vi "Thread Loop.vi"(8 "error in (no error)":errorcluster, 11 "Vehicle Position Simulation in":refnum<class "Vehicle Position Simulation.lvclass">) -> (0 "error out":errorcluster, 3 "Vehicle Position Simulation out":refnum<class "Vehicle Position Simulation.lvclass">)   [LabVIEW 2012, in "Vehicle Position Simulation.lvlib" / "Vehicle Position Simulation.lvclass"]
uses:
  Vehicle Position Simulation.lvclass
  Thread/Thread.lvclass
panel:
  in  "Horizontal Pointer Slide":dbl(slide) scale=0.0..4.0
  # "[Covers: UI4]"
  # "[Covers: UI4A]"
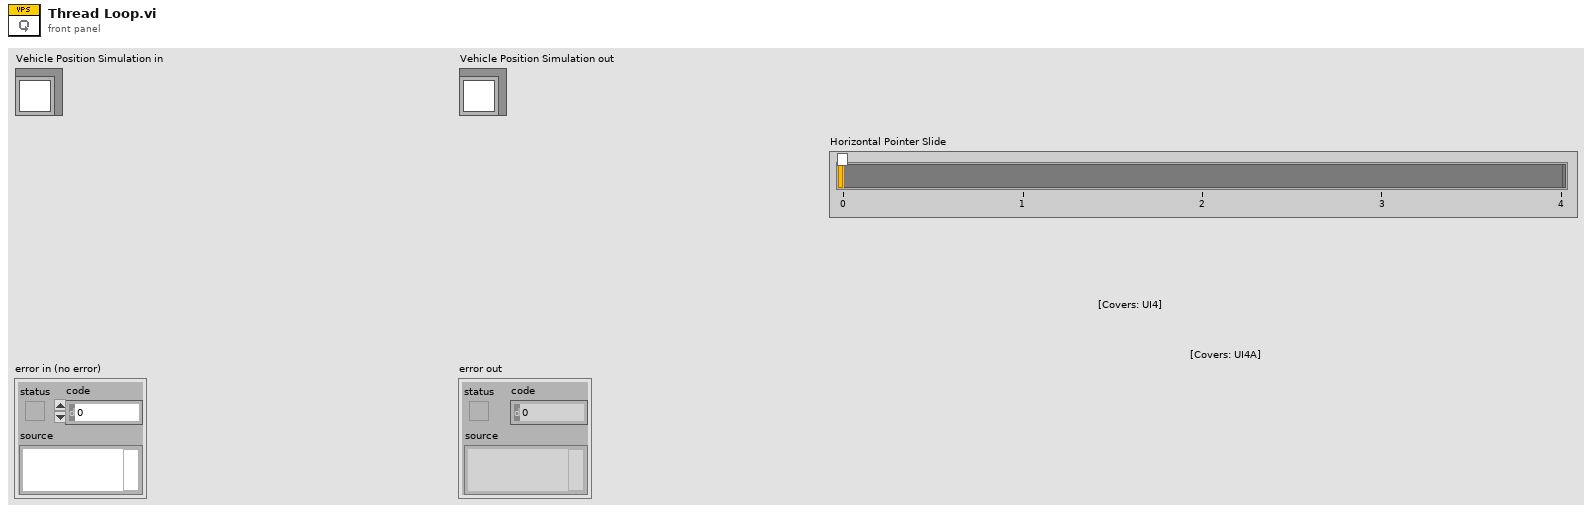
[diagram p1: front panel]
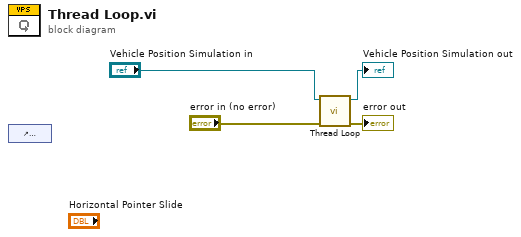
[diagram p0: block diagram]
diagram:
  n1 = control-ref of="Horizontal Pointer Slide"() -> ()  [unwired: 1 out]
  n2 = call-parent "Thread Loop.vi"("error in (no error)"="error in (no error)", "Thread in"="Vehicle Position Simulation in") -> ("error out"=→"error out":errorcluster, "Thread out"=→"Vehicle Position Simulation out":refnum<class "Vehicle Position Simulation.lvclass">)  [unwired: 8 in]
